vi "svi.vi"(11 "x":dbl) -> (3 "new picture":picture)   [LabVIEW 2016]
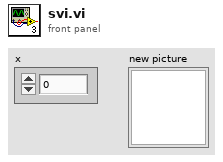
[diagram p1: front panel]
types:
  T1 = cluster{"left":i16, "top":i16, "right":i16, "bottom":i16}
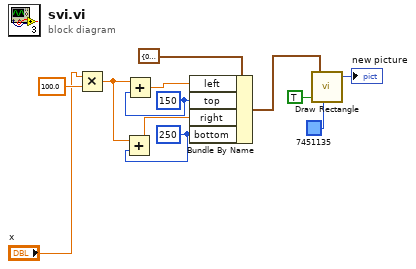
[diagram p0: block diagram]
diagram:
  w9 = i16 250 ("bottom")
  w7 = i16 150 ("top")
  n1 = Multiply(x="x", y=100.0) -> (x*y=w10:dbl)
  n2 = Add(x=w10, y=w9) -> (x+y=w11:dbl)
  n3 = Add(x=w10, y=w7) -> (x+y=w8:dbl)
  n4 = Bundle By Name(cluster=T1 {"left"=0, "top"=0, "right"=0, "bottom"=0} ("rect"), "left"=w8, "top"=w7, "right"=w11, "bottom"=w9) -> (w4:T1)
  n5 = call <vilib>:"Draw Rectangle.vi"("rect"=w4, "fill?(F)"=TRUE, "color(black)"=u32 7451135) -> ("new picture"=→"new picture":picture)  [unwired: 6 in]
